vi "总磷总氮启动参数对话框.vi"() -> (2 "确认":bool, 3 "元素":cluster{"命令":string, "data":variant})   [LabVIEW 2016, in "斯坦道总磷.lvlib"]
panel:
  in  "维护模式":bool=TRUE
  out "标液值":dbl caption="标液值："
  in  "取消":bool
  in  "确定":bool
  in  "量程切换":u16(ring)=2 items=["高量程", "低量程", "自动"]
  in  "站号":u16(ring)=1 items=["总氮"=2, "总磷"=1, "磷酸盐"=4]
  in  "控制命令":T1(ring)
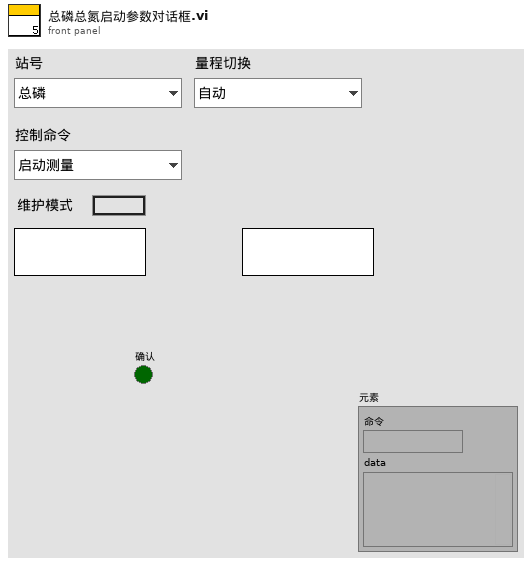
[diagram p1: front panel]
types:
  T1 = enum16{"启动测量", "标样核查", "零点核查", "跨度核查", "空白测试", "平行样测试", "加标回收", "空白校准", "标样校准", "初始化（清洗）", "停止测试", "仪器重启", "校时", "模式设置", "测量间隔设置"}
  T2 = typedef "LVStringsAndValuesArrayTypeDef_U16.ctl" = cluster{"String":string, "Value":u16}[]
  T3 = typedef "操作日志字段定义.ctl" = cluster{"时间":timestamp, "参数":string, "日志信息":string, "流程参数":string}
  T4 = cluster{"站号":u16, "量程切换":enum32{"H", "L", "AUTO"}, "控制命令":enum16{"启动测量", "标样核查", "零点核查", "跨度核查", "空白测试", "平行样测试", "加标回收", "空白校准", "标样校准", "初始化（清洗）", "停止测试", "仪器重启", "校时", "模式设置", "测量间隔设置", "盲样测试"}, "模式设置":enum16{"待机", "连续模式", "周期模式", "定点模式", "受控模式", "手动模式"}, "测量间隔":u16}
  T5 = cluster{"总磷跨度值":dbl, "总磷零点标准液浓度":dbl, "总磷跨度标准液浓度":dbl, "总磷标准液标准浓度":dbl, "总氮跨度值":dbl, "总氮零点标准液浓度":dbl, "总氮跨度标准液浓度":dbl, "总氮标准液标准浓度":dbl, "COD跨度值":dbl, "COD零点标准液浓度":dbl, "COD跨度标准液浓度":dbl, "COD标准液标准浓度":dbl, "氨氮跨度值":dbl, "氨氮零点标准液浓度":dbl, "氨氮跨度标准液浓度":dbl, "氨氮标准液标准浓度":dbl, "磷酸盐跨度值":dbl, "磷酸盐零点标准液浓度":dbl, "磷酸盐跨度标准液浓度":dbl, "磷酸盐标准液标准浓度":dbl, "硝氮跨度值":dbl, "硝氮零点标准液浓度":dbl, "硝氮跨度标准液浓度":dbl, "硝氮标准液标准浓度":dbl, "亚硝氮跨度值":dbl, "亚硝氮零点标准液浓度":dbl, "亚硝氮跨度标准液浓度":dbl, "亚硝氮标准液标准浓度":dbl, "硫化物跨度值":dbl, "硫化物零点标准液浓度":dbl, "硫化物跨度标准液浓度":dbl, "硫化物标准液标准浓度":dbl, "硅酸盐跨度值":dbl, "硅酸盐零点标准液浓度":dbl, "硅酸盐跨度标准液浓度":dbl, "硅酸盐标准液标准浓度":dbl, "总磷零点标准液偏差":dbl, "总磷跨度标准液偏差":dbl, "总磷标准液标准偏差":dbl, "总氮零点标准液偏差":dbl, "总氮跨度标准液偏差":dbl, "总氮标准液标准偏差":dbl, "COD零点标准液偏差":dbl, "COD跨度标准液偏差":dbl, "COD标准液标准偏差":dbl, "氨氮零点标准液偏差":dbl, "氨氮跨度标准液偏差":dbl, "氨氮标准液标准偏差":dbl, "磷酸盐零点标准液偏差":dbl, "磷酸盐跨度标准液偏差":dbl, "磷酸盐标准液标准偏差":dbl, "硝氮零点标准液偏差":dbl, "硝氮跨度标准液偏差":dbl, "硝氮标准液标准偏差":dbl, "亚硝氮零点标准液偏差":dbl, "亚硝氮跨度标准液偏差":dbl, "亚硝氮标准液标准偏差":dbl, "硫化物零点标准液偏差":dbl, "硫化物跨度标准液偏差":dbl, "硫化物标准液标准偏差":dbl, "硅酸盐零点标准液偏差":dbl, "硅酸盐跨度标准液偏差":dbl, "硅酸盐标准液标准偏差":dbl, "氟化物跨度值":dbl, "氟化物零点标准液浓度":dbl, "氟化物跨度标准液浓度":dbl, "氟化物标准液标准浓度":dbl, "氟化物零点标准液偏差":dbl, "氟化物跨度标准液偏差":dbl, "氟化物标准液标准偏差":dbl, "CODMn跨度值":dbl, "CODMn零点标准液浓度":dbl, "CODMn跨度标准液浓度":dbl, "CODMn标准液标准浓度":dbl, "CODMn零点标准液偏差":dbl, "CODMn跨度标准液偏差":dbl, "CODMn标准液标准偏差":dbl}
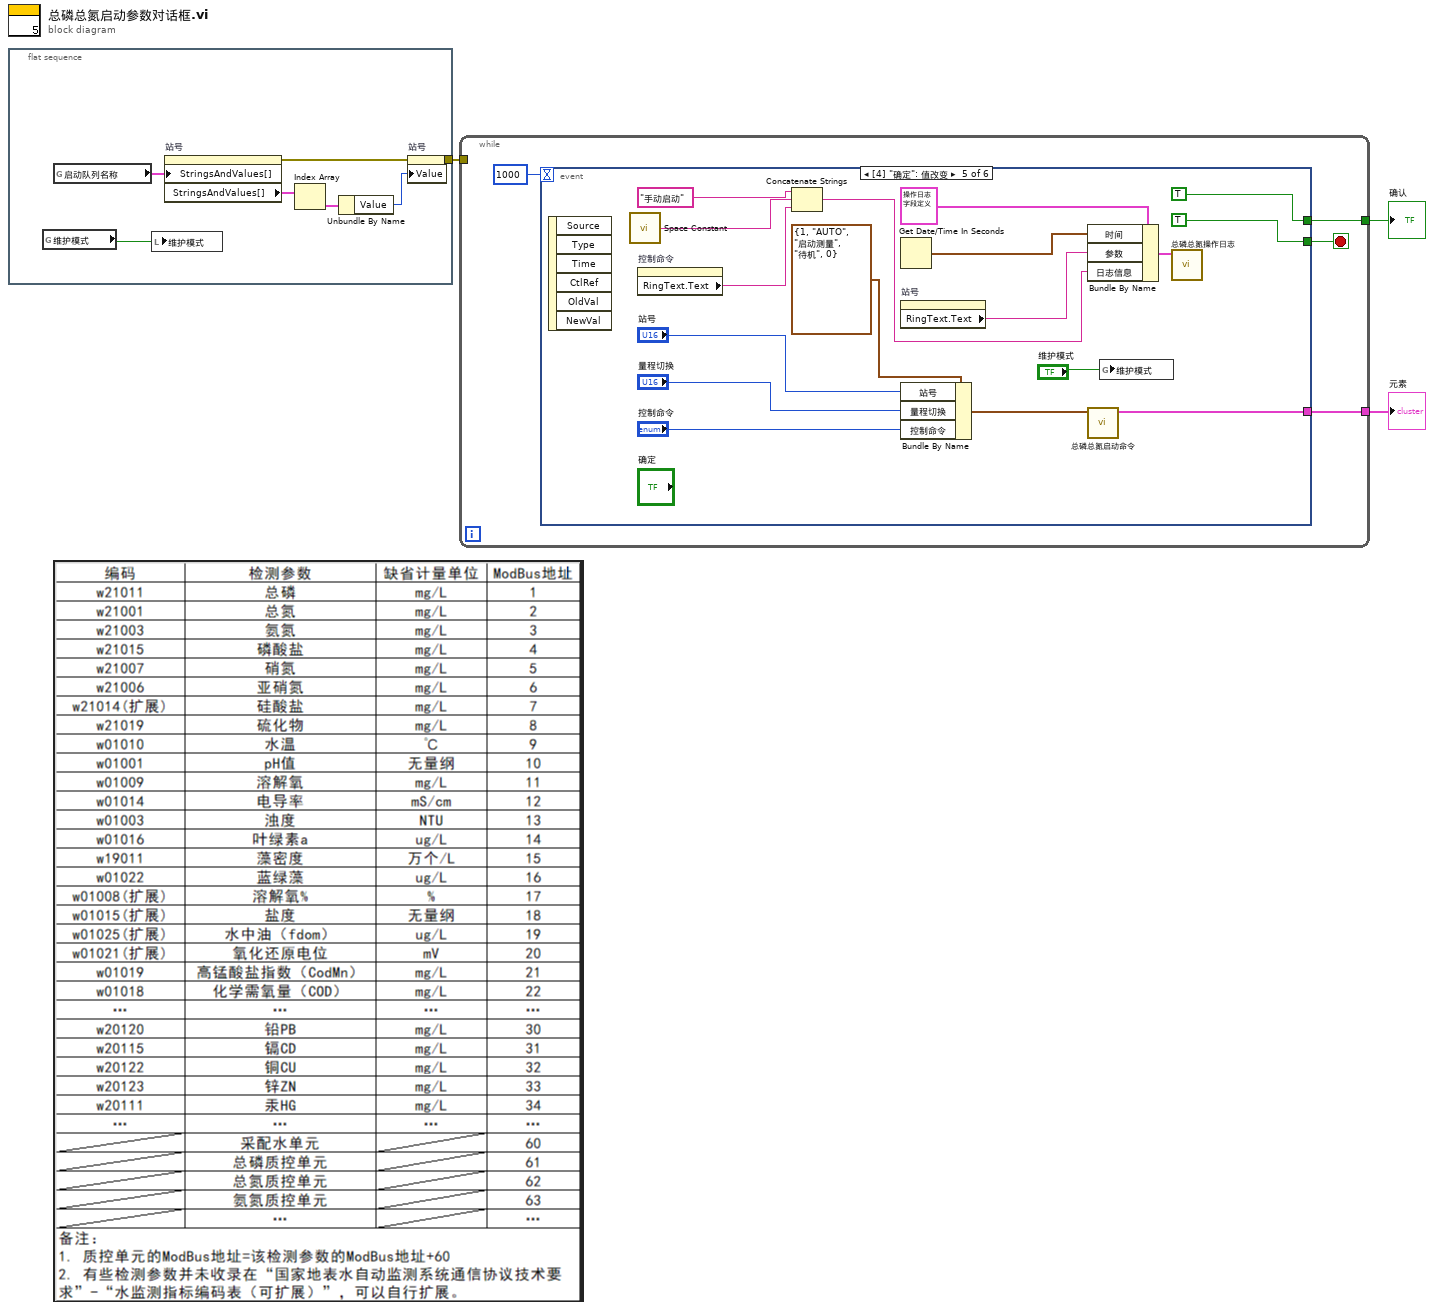
[diagram p0: block diagram]
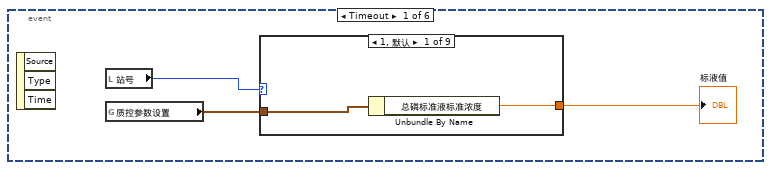
[diagram p2: hidden frame]
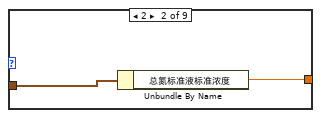
[diagram p3: hidden frame]
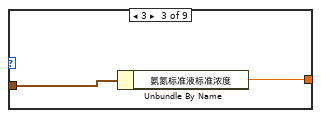
[diagram p4: hidden frame]
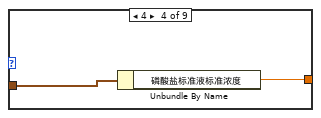
[diagram p5: hidden frame]
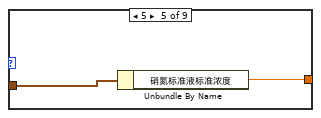
[diagram p6: hidden frame]
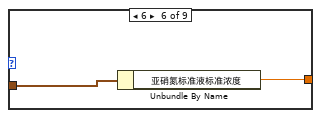
[diagram p7: hidden frame]
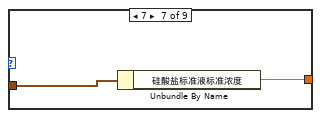
[diagram p8: hidden frame]
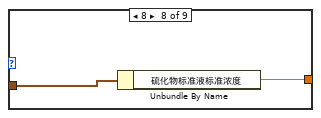
[diagram p9: hidden frame]
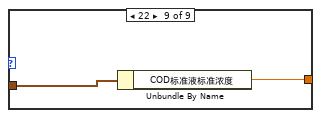
[diagram p10: hidden frame]
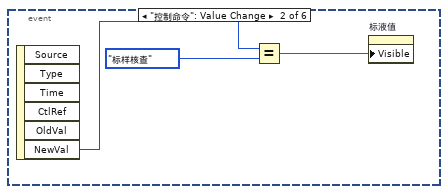
[diagram p11: hidden frame]
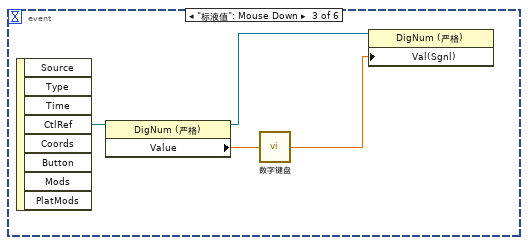
[diagram p12: hidden frame]
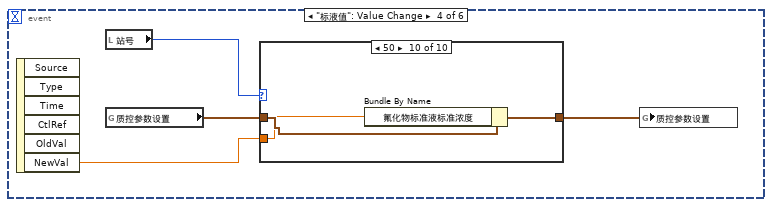
[diagram p13: hidden frame]
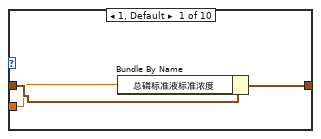
[diagram p14: hidden frame]
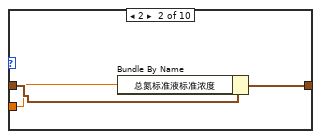
[diagram p15: hidden frame]
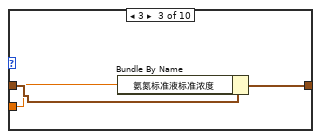
[diagram p16: hidden frame]
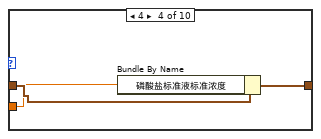
[diagram p17: hidden frame]
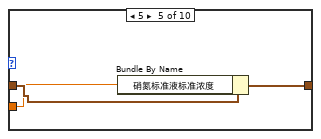
[diagram p18: hidden frame]
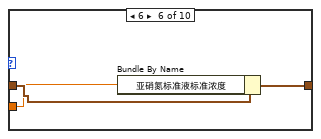
[diagram p19: hidden frame]
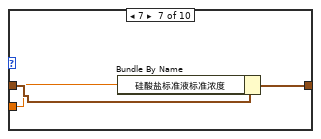
[diagram p20: hidden frame]
diagram:
  n1 = flat-sequence {
    tunnel: [w5] -> w1
    frame #0 {
      n2 = global read "VAR总磷总氮全局变量.vi" "维护模式"() -> (w4:bool)
      n3 = global read "model config var.vi" "启动队列名称"() -> (w10:cluster{"String":string, "Value":u16}[])
      n4 = local write "维护模式"(w4) -> ()
      n5 = property on="站号" class="Ring (严格)"("StringsAndValues[]"=w10) -> (error out=w9:errorcluster, "StringsAndValues[]"=w8:T2)  [unwired: 2 in, 1 out]
      n6 = Index Array(array=w8) -> (element=w7:cluster{"String":string, "Value":u16})  [unwired: 1 in]
      n7 = Unbundle By Name(w7) -> ("Value"=w6:u16)
      n8 = property on="站号" class="Ring (严格)"(error in=w9, "Value"=w6) -> (error out=w5:errorcluster)  [unwired: 1 in, 1 out]
    }
  }
  n9 = while {
    tunnel: [w12] -> w3
    tunnel: [w11] -> w2
    tunnel: w1 -> [_]
    stop <- w14 stop-if-true
    n10 = event shown="[4] \"确定\": 值改变" {
      selector: _ -> [_ _ _ _ _ _]
      dyn-events: _ -> [_ _ _ _ _ _]
      timeout: 1000 -> [_ _ _ _ _ _]
      tunnel: [_ _ _ _ TRUE TRUE] -> w14
      tunnel: [_ _ _ _ TRUE _] -> w12
      tunnel: [_ _ _ _ w91 _] -> w11
      event Timeout {
        n11 = event-data() -> ()  [unwired: 1 in, 3 out]
        n12 = local read "站号"() -> (w16:u16)
        n13 = global read "总磷总氮断电保存全局变量.vi" "质控参数设置"() -> (w17:T5)
        n14 = case shown="1, 默认" w16 {
          tunnel: w17 -> [w19 w21 w23 w25 w27 w29 w31 w33 w35]
          tunnel: [w18 w20 w22 w24 w26 w28 w30 w32 w34] -> w15
          frame 1, Default {
            n15 = Unbundle By Name(w19) -> ("总磷标准液标准浓度"=w18:dbl)
          }
          frame 2 {
            n16 = Unbundle By Name(w21) -> ("总氮标准液标准浓度"=w20:dbl)
          }
          frame 3 {
            n17 = Unbundle By Name(w23) -> ("氨氮标准液标准浓度"=w22:dbl)
          }
          frame 4 {
            n18 = Unbundle By Name(w25) -> ("磷酸盐标准液标准浓度"=w24:dbl)
          }
          frame 5 {
            n19 = Unbundle By Name(w27) -> ("硝氮标准液标准浓度"=w26:dbl)
          }
          frame 6 {
            n20 = Unbundle By Name(w29) -> ("亚硝氮标准液标准浓度"=w28:dbl)
          }
          frame 7 {
            n21 = Unbundle By Name(w31) -> ("硅酸盐标准液标准浓度"=w30:dbl)
          }
          frame 8 {
            n22 = Unbundle By Name(w33) -> ("硫化物标准液标准浓度"=w32:dbl)
          }
          frame 22 {
            n23 = Unbundle By Name(w35) -> ("COD标准液标准浓度"=w34:dbl)
          }
        }
        "标液值" <- w15
      }
      event "控制命令": Value Change {
        n24 = event-data() -> ("NewVal"=w38:T1)  [unwired: 1 in, 5 out]
        n25 = Equal?(x=w38, y=T1."标样核查") -> (x = y?=w36:bool)
        n26 = property on="标液值" class="DigNum (严格)"("Visible"=w36) -> ()  [unwired: 2 in, 2 out]
      }
      event "标液值": Mouse Down {
        n27 = event-data() -> ("CtlRef"=w42:refnum<vi>)  [unwired: 1 in, 7 out]
        n28 = property class="DigNum (严格)"(reference=w42) -> (reference out=w39:refnum<vi>, "Value"=w41:dbl)  [unwired: 1 in, 1 out]
        n29 = call "数字键盘.vi"("OldNumber"=w41) -> ("NewNumber"=w40:dbl)
        n30 = property class="DigNum (严格)"(reference=w39, "Val(Sgnl)"=w40) -> ()  [unwired: 1 in, 2 out]
      }
      event "标液值": Value Change {
        n31 = event-data() -> ("NewVal"=w44:dbl)  [unwired: 1 in, 5 out]
        n32 = local read "站号"() -> (w46:u16)
        n33 = global read "总磷总氮断电保存全局变量.vi" "质控参数设置"() -> (w45:T5)
        n34 = case shown="50" w46 {
          tunnel: w45 -> [w49 w52 w55 w58 w61 w64 w67 w70 w73 w76]
          tunnel: [w47 w50 w53 w56 w59 w62 w65 w68 w71 w74] -> w43
          tunnel: w44 -> [w48 w51 w54 w57 w60 w63 w66 w69 w72 w75]
          frame 1, Default {
            n35 = Bundle By Name(cluster=w49, "总磷标准液标准浓度"=w48) -> (w47:T5)
          }
          frame 2 {
            n36 = Bundle By Name(cluster=w52, "总氮标准液标准浓度"=w51) -> (w50:T5)
          }
          frame 3 {
            n37 = Bundle By Name(cluster=w55, "氨氮标准液标准浓度"=w54) -> (w53:T5)
          }
          frame 4 {
            n38 = Bundle By Name(cluster=w58, "磷酸盐标准液标准浓度"=w57) -> (w56:T5)
          }
          frame 5 {
            n39 = Bundle By Name(cluster=w61, "硝氮标准液标准浓度"=w60) -> (w59:T5)
          }
          frame 6 {
            n40 = Bundle By Name(cluster=w64, "亚硝氮标准液标准浓度"=w63) -> (w62:T5)
          }
          frame 7 {
            n41 = Bundle By Name(cluster=w67, "硅酸盐标准液标准浓度"=w66) -> (w65:T5)
          }
          frame 8 {
            n42 = Bundle By Name(cluster=w70, "硫化物标准液标准浓度"=w69) -> (w68:T5)
          }
          frame 22 {
            n43 = Bundle By Name(cluster=w73, "COD标准液标准浓度"=w72) -> (w71:T5)
          }
          frame 50 {
            n44 = Bundle By Name(cluster=w76, "氟化物标准液标准浓度"=w75) -> (w74:T5)
          }
        }
        n45 = global write "总磷总氮断电保存全局变量.vi" "质控参数设置"(w43) -> ()
      }
      event "确定": Value Change {
        n46 = event-data() -> ()  [unwired: 1 in, 6 out]
        n47 = call <vilib>:"Space Constant.vi"() -> ("String"=w81:string)
        n48 = property on="控制命令" class="Enum (严格)"() -> ("RingText.Text"=w82:string)  [unwired: 2 in, 2 out]
        n49 = Concatenate Strings("手动启动" ("日志信息"), w81, w82) -> (w78:string)
        n50 = Get Date/Time In Seconds() -> (seconds since 1Jan1904=w83:timestamp)
        n51 = property on="站号" class="Ring (严格)"() -> ("RingText.Text"=w80:string)  [unwired: 2 in, 2 out]
        n52 = Bundle By Name(cluster=T4 {"站号"=1, "量程切换"=enum."AUTO", "控制命令"=enum."启动测量", "模式设置"=enum."待机", "测量间隔"=0} ("参数"), "站号"="站号", "量程切换"="量程切换", "控制命令"="控制命令") -> (w89:T4)
        n53 = Bundle By Name(cluster=T3 {"时间"=timestamp(0 s since 1904-01-01), "参数"="", "日志信息"="", "流程参数"=""} ("data in"), "时间"=w83, "参数"=w80, "日志信息"=w78) -> (w84:T3)
        n54 = call "总磷总氮启动命令.vi"("参数"=w89) -> ("启动命令"=w91:cluster{"命令":string, "data":variant})  [unwired: 10 in]
        n55 = global write "VAR总磷总氮全局变量.vi" "维护模式"("维护模式") -> ()
        n56 = call "总磷总氮操作日志.vi"("data in"=w84) -> ()  [unwired: 10 in, 1 out]
      }
      event "取消": Value Change; Panel Close {
        n57 = event-data() -> ()  [unwired: 1 in, 3 out]
      }
    }
  }
  "元素" <- w2
  "确认" <- w3
